vi "Duplicate Control To FP.vi"(8 "error in":errorcluster, 9 "Owner":refnum<vi>, 10 "Control":refnum<vi>) -> (0 "error out":errorcluster)   [LabVIEW 2020, in "_Rescript.lvlib"]
uses:
  _Rescript.lvlib
  <vilib>/Utility/miscctls.llb/LVPositionTypeDef.ctl
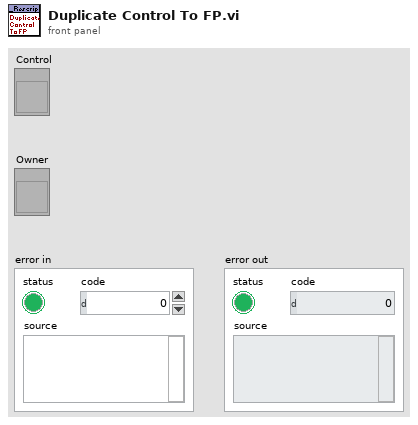
[diagram p1: front panel]
types:
  T1 = typedef "LVPositionTypeDef.ctl" = cluster{"Left":i32, "Top":i32}
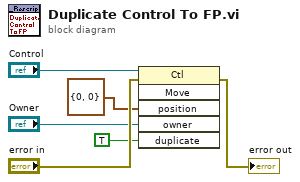
[diagram p0: block diagram]
diagram:
  n1 = invoke class="Ctl" method="Move"(reference="Control", error in="error in", "position"=T1 {"Left"=0, "Top"=0}, "owner"="Owner", "duplicate"=TRUE ("Duplicate? (F)")) -> (error out=→"error out":errorcluster)  [unwired: 1 in, 5 out]
